vi "HexString to HexNum (SubVI).vi"(11 "input string":string) -> (3 "number":u32)   [LabVIEW 2017]
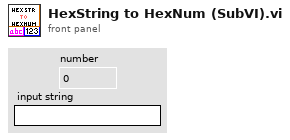
[diagram p1: front panel]
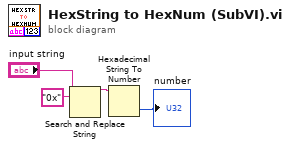
[diagram p0: block diagram]
diagram:
  n1 = Search and Replace String(input string="input string", search string="0x") -> (result string=w4:string)  [unwired: 6 in, 3 out]
  n2 = Hexadecimal String To Number(string=w4) -> (number=→"number":u32)  [unwired: 2 in, 1 out]
